vi "Log View for FFT Spectrum.vi"(2 "channel info":T1={"sensor sensitivity [mV/EU]"=1000.0, "engineering units"=1, "dB reference [EU]"=1.0, "custom label"="EU", "weighting filter"=0, "pregain [dB]"=0.0} {"pregain [dB]" format="%.2f"; "weighting filter" items=["Linear", "A-weighting", "B-weighting", "C-weighting", "ITU-R 468-4", "Dolby", "CCITT", "C-message"]; "dB reference [EU]" format="%^.1e"; "engineering units" items=["custom..."=0, "V"=1, "A"=21, "Pa"=2, "N"=20, "g"=3, "m/s^2"=4, "m/s"=5, "m"=6, "mm/s"=12, "mm"=13, "microns/s"=14, "microns"=15, "in/s^2"=7, "in/s"=8, "in"=9, "mils/s"=10, "mils"=11, "rad/s^2"=16, "rad/s"=17, "rad"=18, "strain"=19]; "sensor sensitivity [mV/EU]" format="%.2f"}, 4 "dB On (T)":bool=TRUE, 5 "FFT spectrum [EUrms]":dbl[](array[numeric]) format="%.2f") -> (0 "unit label":string, 1 "log view FFT spectrum [dB EU]":dbl[](array[numeric]) format="%.2f")   [LabVIEW 2017]
uses:
  <vilib>/addons/Sound and Vibration/compatibility/Controls/svl_Channel Info.ctl
  <vilib>/addons/Sound and Vibration/compatibility/Controls/svl_Engineering Units Text Ring.ctl
  <vilib>/addons/Sound and Vibration/compatibility/Controls/svl_Weighting Filter Text Ring.ctl
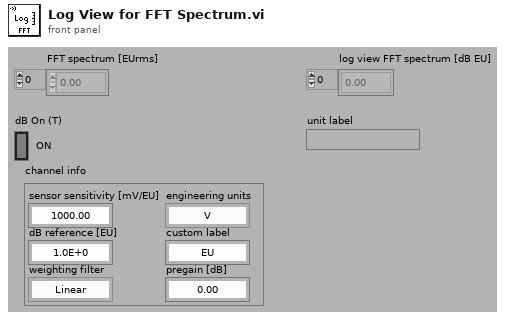
[diagram p1: front panel]
types:
  T1 = typedef "svl_Channel Info.ctl" = cluster{"sensor sensitivity [mV/EU]":dbl, "engineering units":T2, "dB reference [EU]":dbl, "custom label":string, "weighting filter":T3, "pregain [dB]":dbl}
  T2 = typedef "svl_Engineering Units Text Ring.ctl" = u16
  T3 = typedef "svl_Weighting Filter Text Ring.ctl" = u16
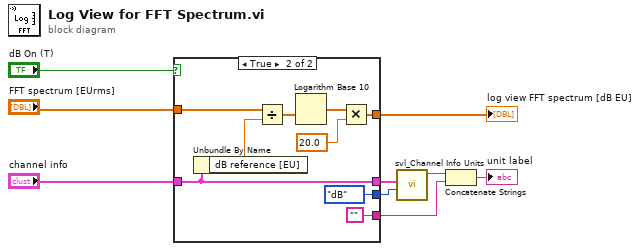
[diagram p0: block diagram]
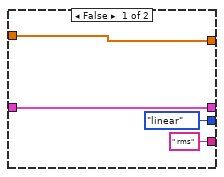
[diagram p2: hidden frame]
diagram:
  n1 = case shown="True" "dB On (T)" {
    tunnel: [w13 w20] -> w6
    tunnel: "channel info" -> [w11 w15]
    tunnel: "FFT spectrum [EUrms]" -> [w13 w19]
    tunnel: [" rms" ""] -> w5
    tunnel: [w11 w15] -> w1
    tunnel: [enum16{"linear", "dB"}."linear" ("linear/dB") enum16{"linear", "dB"}."dB" ("linear/dB")] -> w2
    frame False {
    }
    frame True {
      n2 = Unbundle By Name(w15) -> ("dB reference [EU]"=w17:dbl)
      n3 = Divide(x=w19, y=w17) -> (x/y=w18:dbl[])
      n4 = Logarithm Base 10(1:w18) -> (0:w21:dbl[])
      n5 = Multiply(x=w21, y=20.0) -> (x*y=w20:dbl[])
    }
  }
  "log view FFT spectrum [dB EU]" <- w6
  n6 = call <vilib>:"svl_Channel Info Units.vi"("linear/dB"=w2, "channel info"=w1) -> ("unit label"=w4:string)  [unwired: 8 in, 1 out]
  n7 = Concatenate Strings(w4, w5) -> (→"unit label":string)
